vi "getWIPInfo.vi"(11 "Lotno":string) -> (0 "step":string, 1 "lotno":string, 2 "Package":string, 3 "data":i32, 4 "Product":string, 5 "SSEBATCH":string, 7 "CustomerID":string)   [LabVIEW 2012]
uses:
  <vilib>/addons/database/Auxilliary.llb/DB Tools Cursor Type.ctl
  <vilib>/addons/database/Connection.llb/DB Tools Open Connec (Path).vi
  <vilib>/addons/database/Connection.llb/Conn Execute.vi
  <vilib>/addons/database/Recordset.llb/Rec Fetch Integer Data (R).vi
  <vilib>/addons/database/Recordset.llb/Rec Destroy - Connection.vi
  <vilib>/addons/database/Recordset.llb/Rec Fetch Recordset Data (R).vi
  <vilib>/addons/database/_DB Variant To Data/Database Variant To Data.xnode
  <vilib>/addons/database/NI_Database_API.lvlib
panel:
  out "BATCHQTY":i32
  out "location":string
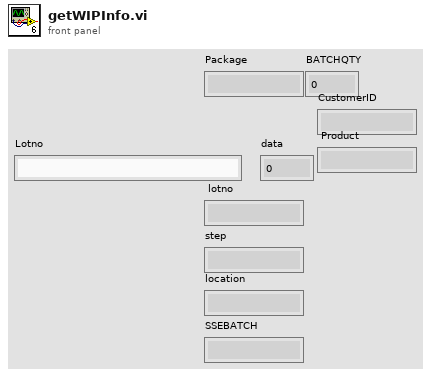
[diagram p1: front panel]
types:
  T1 = typedef "NI_Database_API.lvlib/DB Tools Cursor Type.ctl" = enum16{"forward-only", "keyset", "dynamic", "static"}
  T2 = typedef "NI_Database_API.lvlib/Conn ObjectReference.ctl" = refnum<k1>
  T3 = typedef "NI_Database_API.lvlib/Rec ObjectReference.ctl" = refnum<k1>
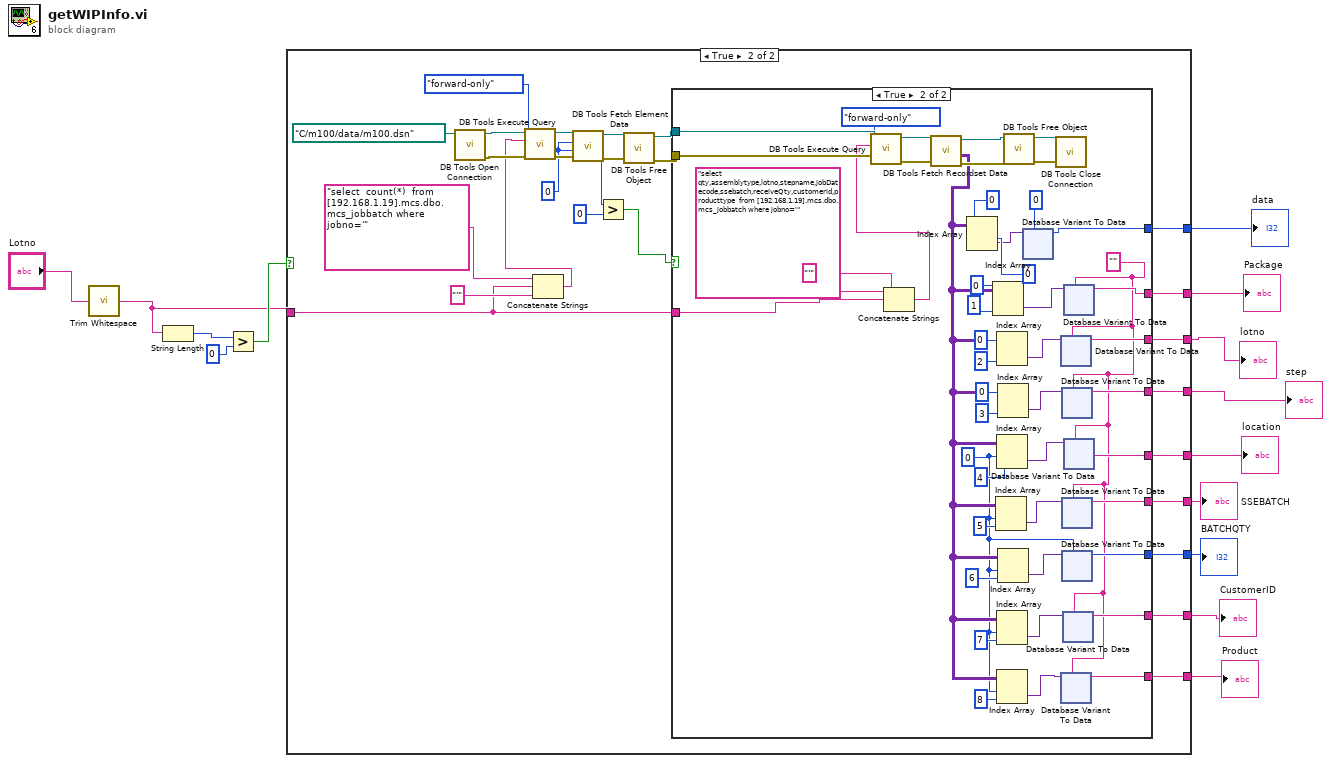
[diagram p0: block diagram]
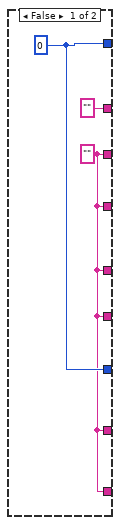
[diagram p2: hidden frame]
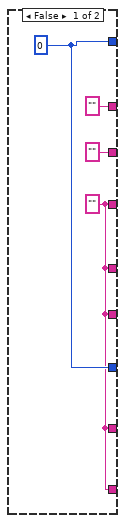
[diagram p3: hidden frame]
diagram:
  n1 = call <vilib>:"Trim Whitespace.vi"("string"="Lotno") -> ("trimmed string"=w1:string)  [unwired: 1 in]
  n2 = String Length(string=w1) -> (length=w14:i32)
  n3 = Greater?(x=w14, y=0) -> (0:w12:bool)
  n4 = case shown="True" w12 {
    tunnel: w1 -> [_ w34]
    tunnel: [w15 w44] -> w11
    tunnel: ["" ("data") w43] -> w10
    tunnel: [w16 w42] -> w9
    tunnel: [w15 w41] -> w8
    tunnel: [w15 w23] -> w7
    tunnel: [w15 w22] -> w6
    tunnel: [w16 w21] -> w5
    tunnel: [w15 w20] -> w4
    tunnel: [w15 w19] -> w3
    frame False {
      w15 = "" ("data")
      w16 = 0 ("data")
    }
    frame True {
      w27 = 0
      n5 = call-poly <vilib>:"DB Tools Open Connection.vi"("connection information"=path "C:/m100/data/m100.dsn") -> ("error out"=w37:errorcluster, "connection reference"=w38:T2)  [unwired: 7 in]
      n6 = Concatenate Strings("select  count(*)  from [192.168.1.19].mcs.dbo.mcs_jobbatch where jobno='" ("string"), w34, "'" ("string")) -> (w32:string)
      n7 = call-poly <vilib>:"DB Tools Execute Query.vi"("error in (no error)"=w37, "cursor type"=DB_Tools_Cursor_Type."forward-only", "SQL query"=w32, "connection reference"=w38) -> ("error out"=w31:errorcluster, "recordset reference"=w30:T3)  [unwired: 4 in]
      n8 = call-poly <vilib>:"DB Tools Fetch Element Data.vi"("error in (no error)"=w31, "type"=w27, "column index"=w27, "recordset reference"=w30) -> ("error out"=w28:errorcluster, "data"=w26:i32, "recordset reference out"=w29:T3)  [unwired: 3 in]
      n9 = Greater?(x=w26, y=0) -> (0:w24:bool)
      n10 = call-poly <vilib>:"DB Tools Free Object.vi"("error in (no error)"=w28, "recordset reference"=w29) -> ("error out"=w39:errorcluster, "connection reference"=w40:T2)  [unwired: 8 in]
      n11 = case shown="True" w24 {
        tunnel: w40 -> [_ w94]
        tunnel: w39 -> [_ w91]
        tunnel: w34 -> [_ w74]
        tunnel: ["" ("data") w73] -> w44
        tunnel: ["" ("data") w72] -> w43
        tunnel: [w46 w71] -> w42
        tunnel: [w45 w67] -> w41
        tunnel: [w45 w64] -> w23
        tunnel: [w45 w59] -> w22
        tunnel: [w46 w58] -> w21
        tunnel: [w45 w55] -> w20
        tunnel: [w45 w49] -> w19
        frame False {
          w45 = "" ("data")
          w46 = 0 ("data")
        }
        frame True {
          w53 = 0 ("index (row)")
          w50 = ""
          n12 = Concatenate Strings("select qty,assemblytype,lotno,stepname,jobDatecode,ssebatch,receiveQty,customerid,producttype  from [192.168.1.19].mcs.dbo.mcs_jobbatch where jobno='" ("string"), w74, "'" ("string")) -> (w85:string)
          n13 = call-poly <vilib>:"DB Tools Execute Query.vi"("error in (no error)"=w91, "cursor type"=DB_Tools_Cursor_Type."forward-only", "SQL query"=w85, "connection reference"=w94) -> ("error out"=w90:errorcluster, "recordset reference"=w93:T3)  [unwired: 4 in]
          n14 = call-poly <vilib>:"DB Tools Fetch Recordset Data.vi"("error in (no error)"=w90, "recordset reference"=w93) -> ("error out"=w89:errorcluster, "recordset data"=w54:variant[][], "recordset reference out"=w92:T3)  [unwired: 3 in]
          n15 = Index Array(array=w54, index (row)=0, index (col)=0 ("disabled index (col)")) -> (element=w82:variant)
          n16 = Index Array(array=w54, index (row)=0 ("disabled index (row)"), index (col)=1 ("disabled index (col)")) -> (element=w78:variant)
          n17 = Index Array(array=w54, index (row)=w53, index (col)=5 ("disabled index (col)")) -> (element=w61:variant)
          n18 = Index Array(array=w54, index (row)=0 ("disabled index (row)"), index (col)=2 ("disabled index (col)")) -> (element=w77:variant)
          n19 = Index Array(array=w54, index (row)=w53, index (col)=4 ("disabled index (col)")) -> (element=w65:variant)
          n20 = Index Array(array=w54, index (row)=w53, index (col)=7 ("disabled index (col)")) -> (element=w56:variant)
          n21 = Index Array(array=w54, index (row)=w53, index (col)=8 ("disabled index (col)")) -> (element=w51:variant)
          n22 = Index Array(array=w54, index (row)=0 ("disabled index (row)"), index (col)=3 ("disabled index (col)")) -> (element=w68:variant)
          n23 = Index Array(array=w54, index (row)=w53, index (col)=6 ("disabled index (col)")) -> (element=w60:variant)
          n24 = call-poly <vilib>:"DB Tools Free Object.vi"("error in (no error)"=w89, "recordset reference"=w92) -> ("error out"=w96:errorcluster, "connection reference"=w95:T2)  [unwired: 8 in]
          n25 = xnode "Database Variant To Data"("database variant"=w82, "type"=0) -> ("data"=w71:i32)  [unwired: 1 in, 1 out]
          n26 = call <vilib>:"DB Tools Close Connection.vi"("error in (no error)"=w96, "connection reference"=w95) -> ()  [unwired: 5 in, 1 out]
          n27 = xnode "Database Variant To Data"("database variant"=w77, "type"=w50) -> ("data"=w73:string)  [unwired: 1 in, 1 out]
          n28 = xnode "Database Variant To Data"("database variant"=w51, "type"=w50) -> ("data"=w49:string)  [unwired: 1 in, 1 out]
          n29 = xnode "Database Variant To Data"("database variant"=w68, "type"=w50) -> ("data"=w67:string)  [unwired: 1 in, 1 out]
          n30 = xnode "Database Variant To Data"("database variant"=w61, "type"=w50) -> ("data"=w59:string)  [unwired: 1 in, 1 out]
          n31 = xnode "Database Variant To Data"("database variant"=w60, "type"=w53) -> ("data"=w58:i32)  [unwired: 1 in, 1 out]
          n32 = xnode "Database Variant To Data"("database variant"=w56, "type"=w50) -> ("data"=w55:string)  [unwired: 1 in, 1 out]
          n33 = xnode "Database Variant To Data"("database variant"=w78, "type"=w50) -> ("data"=w72:string)  [unwired: 1 in, 1 out]
          n34 = xnode "Database Variant To Data"("database variant"=w65, "type"=w50) -> ("data"=w64:string)  [unwired: 1 in, 1 out]
        }
      }
    }
  }
  "data" <- w9
  "Package" <- w10
  "lotno" <- w11
  "step" <- w8
  "location" <- w7
  "SSEBATCH" <- w6
  "BATCHQTY" <- w5
  "CustomerID" <- w4
  "Product" <- w3
